vi "Begin.vi"(8 "error in":errorcluster) -> (0 "error out":errorcluster)   [LabVIEW 2023]
doc: "Called before other user functions, this VI is expected to open initial I/O refnums, load in file data, and do all program initialization. Notice that the <B>error out</B> terminal is simply used for data flow. Wiring it to other structures or subVIs ensures that this VI runs first."
uses:
  <vilib>/Rock Robotics/WPI/DriverStation/WPI_DriverStationRobotMode2.ctl
  <vilib>/Rock Robotics/WPI/Joystick/WPI_JoystickDeviceEnum.ctl
  <vilib>/Rock Robotics/SystemInterfaces/DIO/FPGA_DIOChannel.ctl
  <vilib>/Rock Robotics/WPI/SafetyOutput/WPI_SafetyOutputConfigMenu.ctl
  <vilib>/Rock Robotics/WPI/RobotDrive/WPI_RobotDriveDevRef.ctl
  <vilib>/Rock Robotics/WPI/MotorControl/WPI_MotorControlDeviceRef.ctl
  <vilib>/Rock Robotics/WPI/MotorControl/WPI_MotorControlType.ctl
  <vilib>/Rock Robotics/SystemInterfaces/DIO/FPGA_DIOPWMChannel.ctl
  <vilib>/Rock Robotics/WPI/PWM/WPI_PWMDeadband.ctl
  <vilib>/Rock Robotics/WPI/ThirdParty/REV Robotics/REVLib/Typedef/Spark MAX Motor Type.ctl
  <vilib>/Rock Robotics/WPI/ThirdParty/REV Robotics/REVLib/Typedef/Spark MAX Idle Mode.ctl
  Robot Global Data.vi
  <vilib>/Rock Robotics/Network Tables/NT Write String Array.vi
panel:
  # "Click here to set max"
  # "Click here to set min"
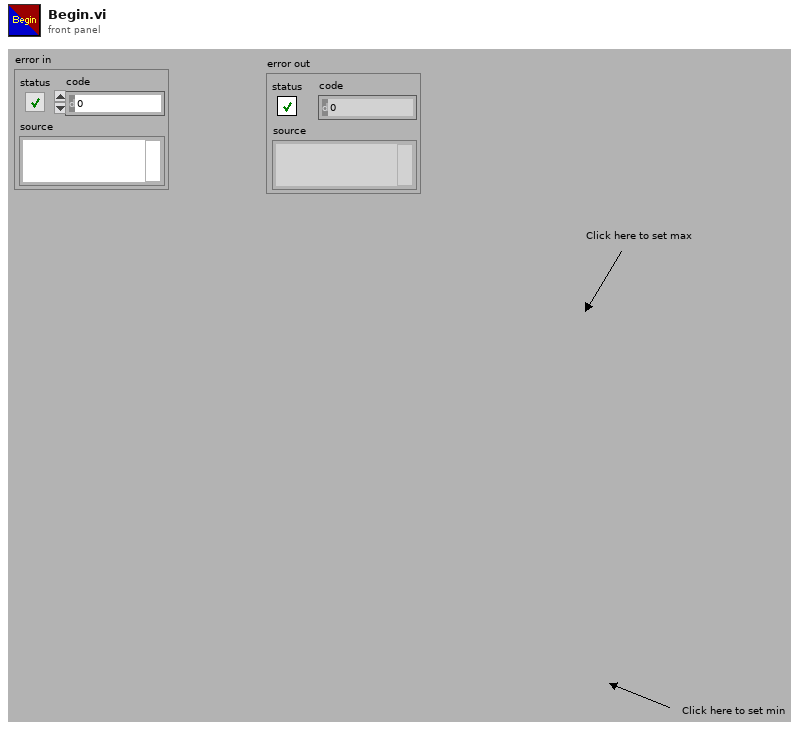
[diagram p1: front panel]
types:
  T1 = typedef "FPGA_DIOChannel.ctl" = enum8{"DIO 0", "DIO 1", "DIO 2", "DIO 3", "DIO 4", "DIO 5", "DIO 6", "DIO 7", "DIO 8", "DIO 9", "DIO MXP 0", "DIO MXP 1", "DIO MXP 2", "DIO MXP 3", "DIO MXP 4", "DIO MXP 5", "DIO MXP 6", "DIO MXP 7", "DIO MXP 8", "DIO MXP 9", "DIO MXP 10", "DIO MXP 11", "DIO MXP 12", "DIO MXP 13", "DIO MXP 14", "DIO MXP 15", "SPI Port CS1", "SPI Port CS2", "SPI Port CS3", "SPI Port MISO", "SPI Port MOSI", "Invalid"}
  T2 = typedef "Spark MAX Idle Mode.ctl" = enum16{"Coast", "Brake"}
  T3 = typedef "Spark MAX Motor Type.ctl" = enum16{"Brushed", "Brushless"}
  T4 = typedef "WPI_JoystickDeviceEnum.ctl" = enum16{"USB 0", "USB 1", "USB 2", "USB 3", "USB 4", "USB 5"}
  T5 = typedef "WPI_RobotDriveDevRef.ctl" = cluster{"DevStatus":errorcluster, "Motors[]":T6[], "Square Inputs":bool, "Max Output":dbl}
  T6 = typedef "WPI_MotorControlDeviceRef.ctl" = cluster{"DeviceStatus":errorcluster, "Type":T7, "PWM":cluster{"PWM Channel":T8, "DeadBand":T9}, "CAN":cluster{"Device Number":u8, "SetOutput VI Ref":variant, "GetOutput VI Ref":variant, "Enable VI Ref":variant, "Disable VI Ref":variant, "Data":variant}, "Invert":bool, "DIO PWM":cluster{"PWM \"Enable\" Channel":T8, "DIOChannel":T1, "PWM Rate":dbl}}
  T7 = typedef "WPI_MotorControlType.ctl" = enum16{"PWM", "CAN", "DIO PWM"}
  T8 = typedef "FPGA_DIOPWMChannel.ctl" = enum8{"PWM 0", "PWM 1", "PWM 2", "PWM 3", "PWM 4", "PWM 5", "PWM 6", "PWM 7", "PWM 8", "PWM 9", "PWM MXP 0", "PWM MXP 1", "PWM MXP 2", "PWM MXP 3", "PWM MXP 4", "PWM MXP 5", "PWM MXP 6", "PWM MXP 7", "PWM MXP 8", "PWM MXP 9", "Invalid"}
  T9 = typedef "WPI_PWMDeadband.ctl" = cluster{"Name":string, "maxPositivePwm":i32, "minPositivePwm":i32, "centerPwm":i32, "maxNegativePwm":i32, "minNegativePwm":i32, "angularRange":u16}
  T10 = typedef "WPI_SafetyOutputConfigMenu.ctl" = enum16{"Enable", "Disable"}
  T11 = typedef "WPI_DriverStationRobotMode2.ctl" = enum16{"Autonomous Disabled", "Autonomous Enabled", "Teleop Disabled", "Teleop Enabled", "Disconnected", "Finish", "Test Disabled", "Test Enabled", "Emergency Stopped"}
  T12 = typedef "WPI_JoystickDevRef.ctl" = cluster{"Device":T4}
  T13 = typedef "WPI_DigitalInputDevRef.ctl" = cluster{"DevStatus":errorcluster, "DIO Channel":T1}
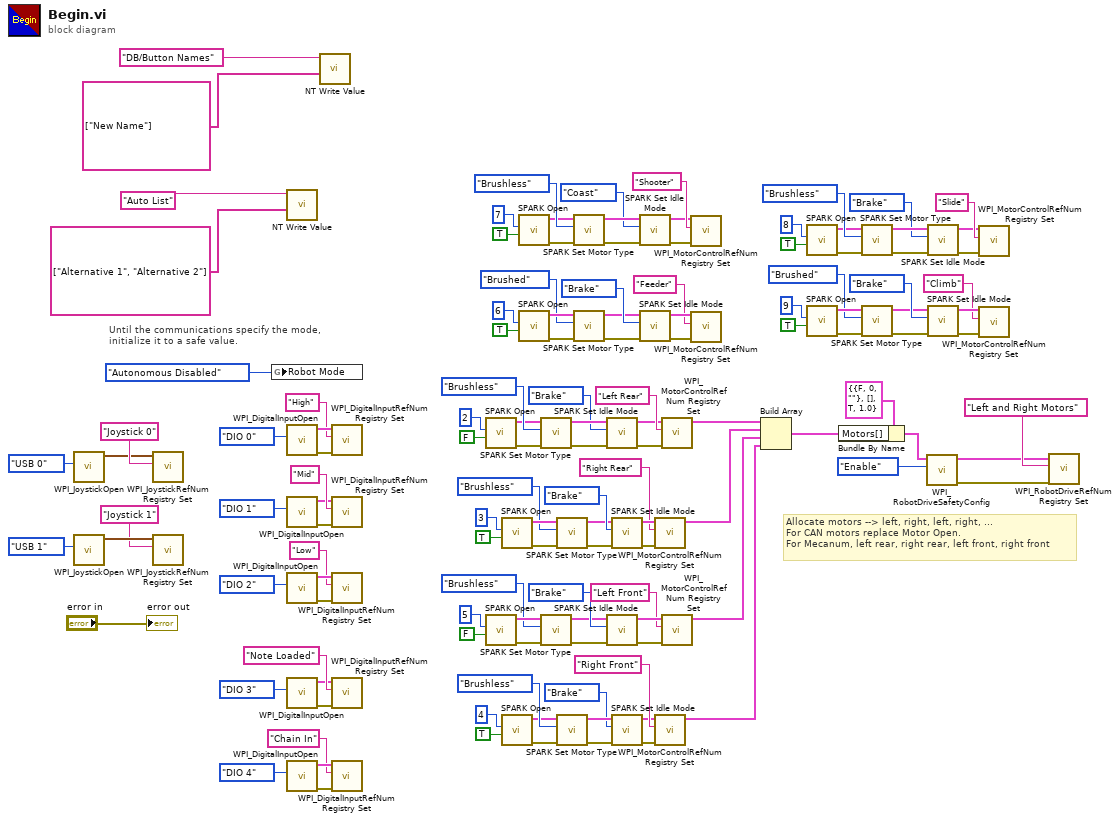
[diagram p0: block diagram]
diagram:
  # "Allocate motors --> left, right, left, right, ... \nFor CAN motors replace Motor Open.\nFor Mecanum, left rear, right rear, left front, right front"
  # "Until the communications specify the mode,\ninitialize it to a safe value."
  n1 = call <vilib>:"WPI_JoystickOpen.vi"("JoystickDevice"=WPI_JoystickDeviceEnum."USB 0") -> ("JoystickDevRef"=w128:T12)  [unwired: 10 in]
  n2 = call <vilib>:"WPI_JoystickOpen.vi"("JoystickDevice"=WPI_JoystickDeviceEnum."USB 1") -> ("JoystickDevRef"=w21:T12)  [unwired: 10 in]
  n3 = call <vilib>:"WPI_JoystickRefNum Registry Set.vi"("refnum name"="Joystick 0", "JoystickDevRef"=w128) -> ()  [unwired: 8 in, 2 out]
  n4 = call <vilib>:"WPI_JoystickRefNum Registry Set.vi"("refnum name"="Joystick 1", "JoystickDevRef"=w21) -> ()  [unwired: 8 in, 2 out]
  n5 = global write "Robot Global Data.vi" "Robot Mode"(WPI_DriverStationRobotMode2."Autonomous Disabled" ("Robot Mode")) -> ()
  n6 = call-poly <vilib>:"NT Write Value.vi"("value"=string[] ["Alternative 1", "Alternative 2"] ("String Array"), "name"="Auto List" ("Name")) -> ()  [unwired: 9 in, 1 out]
  n7 = call <vilib>:"WPI_DigitalInputOpen.vi"("DIO Channel"=FPGA_DIOChannel."DIO 0") -> ("error out"=w119:errorcluster, "DigitalInputDevRef"=w120:T13)  [unwired: 9 in]
  n8 = call <vilib>:"WPI_DigitalInputOpen.vi"("DIO Channel"=FPGA_DIOChannel."DIO 1") -> ("error out"=w116:errorcluster, "DigitalInputDevRef"=w115:T13)  [unwired: 9 in]
  n9 = call <vilib>:"WPI_DigitalInputOpen.vi"("DIO Channel"=FPGA_DIOChannel."DIO 2") -> ("error out"=w111:errorcluster, "DigitalInputDevRef"=w112:T13)  [unwired: 9 in]
  n10 = call <vilib>:"WPI_DigitalInputOpen.vi"("DIO Channel"=FPGA_DIOChannel."DIO 3") -> ("error out"=w7:errorcluster, "DigitalInputDevRef"=w6:T13)  [unwired: 9 in]
  n11 = call <vilib>:"WPI_DigitalInputOpen.vi"("DIO Channel"=FPGA_DIOChannel."DIO 4") -> ("error out"=w2:errorcluster, "DigitalInputDevRef"=w3:T13)  [unwired: 9 in]
  n12 = call-poly <vilib>:"NT Write Value.vi"("value"=string[] ["New Name"], "name"="DB/Button Names" ("Name")) -> ()  [unwired: 9 in, 1 out]
  n13 = call <vilib>:"WPI_DigitalInputRefNum Registry Set.vi"("error in (no error)"=w119, "refnum name"="High", "DigitalInputDevRef"=w120) -> ()  [unwired: 7 in, 2 out]
  n14 = call <vilib>:"WPI_DigitalInputRefNum Registry Set.vi"("error in (no error)"=w116, "refnum name"="Mid", "DigitalInputDevRef"=w115) -> ()  [unwired: 7 in, 2 out]
  n15 = call <vilib>:"WPI_DigitalInputRefNum Registry Set.vi"("error in (no error)"=w111, "refnum name"="Low", "DigitalInputDevRef"=w112) -> ()  [unwired: 7 in, 2 out]
  n16 = call <vilib>:"WPI_DigitalInputRefNum Registry Set.vi"("error in (no error)"=w7, "refnum name"="Note Loaded", "DigitalInputDevRef"=w6) -> ()  [unwired: 7 in, 2 out]
  n17 = call <vilib>:"WPI_DigitalInputRefNum Registry Set.vi"("error in (no error)"=w2, "refnum name"="Chain In", "DigitalInputDevRef"=w3) -> ()  [unwired: 7 in, 2 out]
  n18 = call <vilib>:"SPARK Open.vi"("Invert"=FALSE, "Device Number"=u8 2) -> ("error out"=w102:errorcluster, "MotorControlDeviceRef"=w103:T6)  [unwired: 8 in]
  n19 = call <vilib>:"SPARK Open.vi"("Invert"=FALSE, "Device Number"=u8 5) -> ("error out"=w63:errorcluster, "MotorControlDeviceRef"=w62:T6)  [unwired: 8 in]
  n20 = call <vilib>:"SPARK Open.vi"("Invert"=TRUE, "Device Number"=u8 3) -> ("error out"=w85:errorcluster, "MotorControlDeviceRef"=w84:T6)  [unwired: 8 in]
  n21 = call <vilib>:"SPARK Open.vi"("Invert"=TRUE, "Device Number"=u8 4) -> ("error out"=w80:errorcluster, "MotorControlDeviceRef"=w81:T6)  [unwired: 8 in]
  n22 = call <vilib>:"SPARK Open.vi"("Invert"=TRUE, "Device Number"=u8 7) -> ("error out"=w39:errorcluster, "MotorControlDeviceRef"=w40:T6)  [unwired: 8 in]
  n23 = call <vilib>:"SPARK Open.vi"("Invert"=TRUE, "Device Number"=u8 6) -> ("error out"=w50:errorcluster, "MotorControlDeviceRef"=w49:T6)  [unwired: 8 in]
  n24 = call <vilib>:"SPARK Set Motor Type.vi"("error in (no error)"=w102, "Motor Type"=Spark_MAX_Motor_Type."Brushless", "MotorControlDevRef"=w103) -> ("error out"=w98:errorcluster, "MotorControlDeviceRef"=w99:T6)  [unwired: 7 in]
  n25 = call <vilib>:"SPARK Set Motor Type.vi"("error in (no error)"=w63, "Motor Type"=Spark_MAX_Motor_Type."Brushless", "MotorControlDevRef"=w62) -> ("error out"=w67:errorcluster, "MotorControlDeviceRef"=w66:T6)  [unwired: 7 in]
  n26 = call <vilib>:"SPARK Set Motor Type.vi"("error in (no error)"=w85, "Motor Type"=Spark_MAX_Motor_Type."Brushless", "MotorControlDevRef"=w84) -> ("error out"=w89:errorcluster, "MotorControlDeviceRef"=w88:T6)  [unwired: 7 in]
  n27 = call <vilib>:"SPARK Set Motor Type.vi"("error in (no error)"=w80, "Motor Type"=Spark_MAX_Motor_Type."Brushless", "MotorControlDevRef"=w81) -> ("error out"=w76:errorcluster, "MotorControlDeviceRef"=w77:T6)  [unwired: 7 in]
  n28 = call <vilib>:"SPARK Set Motor Type.vi"("error in (no error)"=w39, "Motor Type"=Spark_MAX_Motor_Type."Brushless", "MotorControlDevRef"=w40) -> ("error out"=w35:errorcluster, "MotorControlDeviceRef"=w36:T6)  [unwired: 7 in]
  n29 = call <vilib>:"SPARK Set Motor Type.vi"("error in (no error)"=w50, "Motor Type"=Spark_MAX_Motor_Type."Brushed", "MotorControlDevRef"=w49) -> ("error out"=w54:errorcluster, "MotorControlDeviceRef"=w53:T6)  [unwired: 7 in]
  n30 = call <vilib>:"SPARK Set Idle Mode.vi"("error in (no error)"=w98, "Idle Mode"=Spark_MAX_Idle_Mode."Brake", "MotorControlDeviceRef in"=w99) -> ("error out"=w94:errorcluster, "MotorControlDeviceRef out"=w95:T6)  [unwired: 7 in]
  n31 = call <vilib>:"SPARK Set Idle Mode.vi"("error in (no error)"=w67, "Idle Mode"=Spark_MAX_Idle_Mode."Brake", "MotorControlDeviceRef in"=w66) -> ("error out"=w71:errorcluster, "MotorControlDeviceRef out"=w70:T6)  [unwired: 7 in]
  n32 = call <vilib>:"SPARK Set Idle Mode.vi"("error in (no error)"=w89, "Idle Mode"=Spark_MAX_Idle_Mode."Brake", "MotorControlDeviceRef in"=w88) -> ("error out"=w93:errorcluster, "MotorControlDeviceRef out"=w92:T6)  [unwired: 7 in]
  n33 = call <vilib>:"SPARK Set Idle Mode.vi"("error in (no error)"=w76, "Idle Mode"=Spark_MAX_Idle_Mode."Brake", "MotorControlDeviceRef in"=w77) -> ("error out"=w72:errorcluster, "MotorControlDeviceRef out"=w73:T6)  [unwired: 7 in]
  n34 = call <vilib>:"SPARK Set Idle Mode.vi"("error in (no error)"=w35, "Idle Mode"=Spark_MAX_Idle_Mode."Coast", "MotorControlDeviceRef in"=w36) -> ("error out"=w42:errorcluster, "MotorControlDeviceRef out"=w43:T6)  [unwired: 7 in]
  n35 = call <vilib>:"SPARK Set Idle Mode.vi"("error in (no error)"=w54, "Idle Mode"=Spark_MAX_Idle_Mode."Brake", "MotorControlDeviceRef in"=w53) -> ("error out"=w47:errorcluster, "MotorControlDeviceRef out"=w46:T6)  [unwired: 7 in]
  n36 = call <vilib>:"WPI_MotorControlRefNum Registry Set.vi"("error in (no error)"=w93, "refnum name"="Right Rear", "MotorControlDevRef"=w92) -> ("MotorControlDevRef"=w59:T6)  [unwired: 7 in, 1 out]
  n37 = call <vilib>:"WPI_MotorControlRefNum Registry Set.vi"("error in (no error)"=w72, "refnum name"="Right Front", "MotorControlDevRef"=w73) -> ("MotorControlDevRef"=w57:T6)  [unwired: 7 in, 1 out]
  n38 = call <vilib>:"WPI_MotorControlRefNum Registry Set.vi"("error in (no error)"=w94, "refnum name"="Left Rear", "MotorControlDevRef"=w95) -> ("MotorControlDevRef"=w60:T6)  [unwired: 7 in, 1 out]
  n39 = call <vilib>:"WPI_MotorControlRefNum Registry Set.vi"("error in (no error)"=w71, "refnum name"="Left Front", "MotorControlDevRef"=w70) -> ("MotorControlDevRef"=w58:T6)  [unwired: 7 in, 1 out]
  n40 = call <vilib>:"WPI_MotorControlRefNum Registry Set.vi"("error in (no error)"=w42, "refnum name"="Shooter", "MotorControlDevRef"=w43) -> ()  [unwired: 7 in, 2 out]
  n41 = call <vilib>:"WPI_MotorControlRefNum Registry Set.vi"("error in (no error)"=w47, "refnum name"="Feeder", "MotorControlDevRef"=w46) -> ()  [unwired: 7 in, 2 out]
  n42 = Build Array(w60, w59, w58, w57) -> (w56:T6[])
  n43 = call <vilib>:"SPARK Open.vi"("Invert"=TRUE, "Device Number"=u8 8) -> ("error out"=w28:errorcluster, "MotorControlDeviceRef"=w29:T6)  [unwired: 8 in]
  n44 = call <vilib>:"SPARK Open.vi"("Invert"=TRUE, "Device Number"=u8 9) -> ("error out"=w14:errorcluster, "MotorControlDeviceRef"=w13:T6)  [unwired: 8 in]
  n45 = Bundle By Name(cluster=T5 {"DevStatus"={"status"=FALSE, "code"=0, "source"=""}, "Motors[]"=[], "Square Inputs"=TRUE, "Max Output"=1.0} ("RobotDriveDevRef"), "Motors[]"=w56) -> (w109:T5)
  n46 = call <vilib>:"SPARK Set Motor Type.vi"("error in (no error)"=w28, "Motor Type"=Spark_MAX_Motor_Type."Brushless", "MotorControlDevRef"=w29) -> ("error out"=w24:errorcluster, "MotorControlDeviceRef"=w25:T6)  [unwired: 7 in]
  n47 = call <vilib>:"SPARK Set Motor Type.vi"("error in (no error)"=w14, "Motor Type"=Spark_MAX_Motor_Type."Brushed", "MotorControlDevRef"=w13) -> ("error out"=w18:errorcluster, "MotorControlDeviceRef"=w17:T6)  [unwired: 7 in]
  n48 = call <vilib>:"WPI_RobotDriveSafetyConfig.vi"("mode"=WPI_SafetyOutputConfigMenu."Enable", "RobotDriveDevRef"=w109) -> ("error out"=w105:errorcluster, "RobotDriveDevRef"=w106:T5)  [unwired: 2 in, 6 out]
  n49 = call <vilib>:"SPARK Set Idle Mode.vi"("error in (no error)"=w24, "Idle Mode"=Spark_MAX_Idle_Mode."Brake", "MotorControlDeviceRef in"=w25) -> ("error out"=w31:errorcluster, "MotorControlDeviceRef out"=w32:T6)  [unwired: 7 in]
  n50 = call <vilib>:"SPARK Set Idle Mode.vi"("error in (no error)"=w18, "Idle Mode"=Spark_MAX_Idle_Mode."Brake", "MotorControlDeviceRef in"=w17) -> ("error out"=w11:errorcluster, "MotorControlDeviceRef out"=w10:T6)  [unwired: 7 in]
  n51 = call <vilib>:"WPI_MotorControlRefNum Registry Set.vi"("error in (no error)"=w31, "refnum name"="Slide", "MotorControlDevRef"=w32) -> ()  [unwired: 7 in, 2 out]
  n52 = call <vilib>:"WPI_MotorControlRefNum Registry Set.vi"("error in (no error)"=w11, "refnum name"="Climb", "MotorControlDevRef"=w10) -> ()  [unwired: 7 in, 2 out]
  n53 = call <vilib>:"WPI_RobotDriveRefNum Registry Set.vi"("error in (no error)"=w105, "refnum name"="Left and Right Motors", "RobotDriveDevRef"=w106) -> ()  [unwired: 1 in, 8 out]
  "error out" <- "error in"
